vi "mxwScript_Cmnd2Str_setLVSpecificPathInfo.vi"(8 "error in (no error)":errorcluster, 11 "data":variant) -> (0 "error out":errorcluster, 3 "outputString":string)   [LabVIEW 2017]
uses:
  codeGenAPISupport.llb/cgAPI_mxwScript_OpenTempl_LabVIEWSpecificPathInfo.ctl
  codeGenAPISupport.llb/cgAPI_mxwScript_OpenTempl_PathGenerationType.ctl
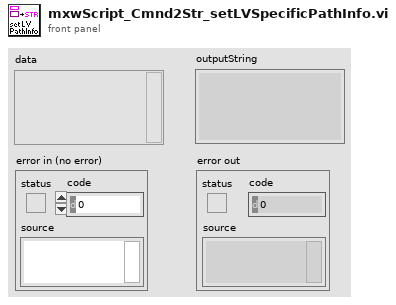
[diagram p1: front panel]
types:
  T1 = typedef "cgAPI_mxwScript_OpenTempl_LabVIEWSpecificPathInfo.ctl" = cluster{"pathGenerationType":T2, "locationIndex":i32, "locationName":string, "pathFormat":string, "useVersionIncrement":bool}
  T2 = typedef "cgAPI_mxwScript_OpenTempl_PathGenerationType.ctl" = enum16{"IndexFromEnd", "Name", "BeforeLLB"}
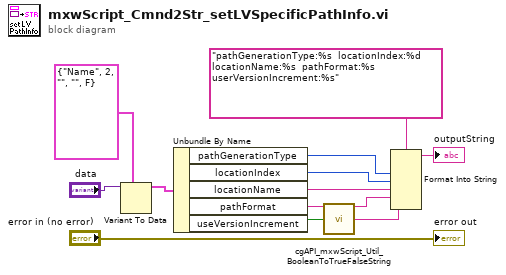
[diagram p0: block diagram]
diagram:
  n1 = Variant To Data(type=T1 {"pathGenerationType"=enum."Name", "locationIndex"=2, "locationName"="", "pathFormat"="", "useVersionIncrement"=FALSE} ("LabVIEWSpecificPath data"), Variant="data") -> (data=w10:T1)  [unwired: 1 in, 1 out]
  n2 = Unbundle By Name(w10) -> ("pathGenerationType"=w5:T2, "locationIndex"=w4:i32, "locationName"=w3:string, "pathFormat"=w2:string, "useVersionIncrement"=w7:bool)
  n3 = call "cgAPI_mxwScript_Util_BooleanToTrueFalseString.vi"("boolean"=w7) -> ("TRUE/FALSE text"=w6:string)  [unwired: 4 out]
  n4 = Format Into String(format string="pathGenerationType:%s  locationIndex:%d  locationName:%s  pathFormat:%s  userVersionIncrement:%s", w5, w4, w3, w2, w6) -> (resulting string=→"outputString":string)  [unwired: 2 in, 1 out]
  "error out" <- "error in (no error)"
